vi "Stop.vi"(8 "error in (no error)":errorcluster, 10 "Address (1)":u16=1 max=15 step=1, 11 "VISA resource name":refnum<visa-resource-name>) -> (0 "error out":errorcluster, 3 "VISA resource name out":refnum<visa-resource-name>)   [LabVIEW 2021, in "Copy of Kloehn V6 Series.lvlib"]
doc: "Halts whatever operation the syringe pump is currently carrying out."
uses:
  Copy of Kloehn V6 Series.lvlib
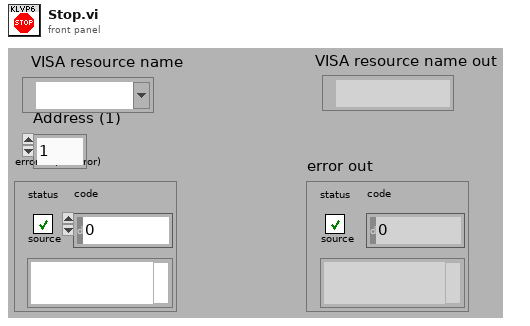
[diagram p1: front panel]
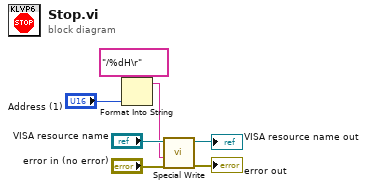
[diagram p0: block diagram]
diagram:
  n1 = Format Into String(format string="/%dH\r", "Address (1)") -> (resulting string=w1:string)  [unwired: 2 in, 1 out]
  n2 = call "Special Write.vi"("error in (no error)"="error in (no error)", "Send String"=w1, "VISA resource name"="VISA resource name") -> ("error out"=→"error out":errorcluster, "VISA resource name out"=→"VISA resource name out":refnum<visa-resource-name>)  [unwired: 4 in, 3 out]
